vi "Asynchronous - Update Disable Channels.vi"(5 "Channel Data []":T3[](array[typedef])=[{"Labels Settings"=[{"Name"="", "xmlName"="", "Label"=0, "transferPeriod"=0, "SDI_Enabled"=FALSE, "SDI"=0, "Word"={"Param Setting"={"Start Bit"=[], "Num Bits"=[], "Signed?"=[], "ScaleFac"=[], "ScaleOffset"=[], "Block Data Refs"=[], "Encoding"=[], "Values Array"=[], "Item Refs"=[]}}, "TransferType"=enum."ScheduledLabel", "has timestamp?"=FALSE, "Label Disable/Trigger Channel Reference"=0, "Message Handle"=0, "Initialized?"=FALSE, "Word Initial Raw Value"=0, "Label Timestamp Channel Data Reference"=0}], "channel handle"=0, "channel #"=0}] {"Labels Settings"."Label Timestamp Channel Data Reference" format="%.0x"; "Labels Settings"."Label Disable/Trigger Channel Reference" format="%.0x"; "Labels Settings"."Word"."Param Setting"."Item Refs" format="%.0x"; "Labels Settings"."Word"."Param Setting"."Num Bits" min=1 max=32; "Labels Settings"."Word"."Param Setting"."Start Bit" min=8 max=31; "Labels Settings"."Label" format="%.0o"}, 7 "Map":T1[](array[typedef]) {"Channel Data Reference" format="%.0x"}, 8 "Error (in)":errorcluster, 9 "Updated FIFO Index []":i32[](array[numeric]), 10 "Doubles []":dbl[](array[numeric])) -> (0 "Error (out)":errorcluster)   [LabVIEW 2020, in "Ballard Arinc-429 Engine.lvlib"]
uses:
  Ballard Arinc-429 Engine.lvlib
  Shared/Controls and Global/RT HW Channel.ctl
  Shared/Controls and Global/RT Label Settings.ctl
  Shared/Controls and Global/Label.ctl
  Shared/Controls and Global/transferPeriod.ctl
  Shared/Controls and Global/RT Word Settings.ctl
  Shared/Controls and Global/RT Param Setting.ctl
  Shared/Controls and Global/Start Bit.ctl
  Shared/Controls and Global/Number of Bits.ctl
  <vilib>/NI VeriStand/Custom Device API/Block Data Reference.ctl
  <vilib>/NI VeriStand/Custom Device API/Data Reference.ctl
  <vilib>/NI VeriStand/Custom Device API/Custom Device Item Ref.ctl
  Shared/Controls and Global/TransferType.ctl
  RT Controls/RT Tx Association.ctl
  <instrlib>/BTI429Lib/BTI429LV.lvlib
  <vilib>/NI VeriStand/Custom Device Tools/Custom Device Utility Library/Custom Device Utility Library.lvlib
  Shared/Ballard Arinc-429 Shared.lvlib
  <vilib>/NI VeriStand/Custom Device API/Custom Device API.lvlib
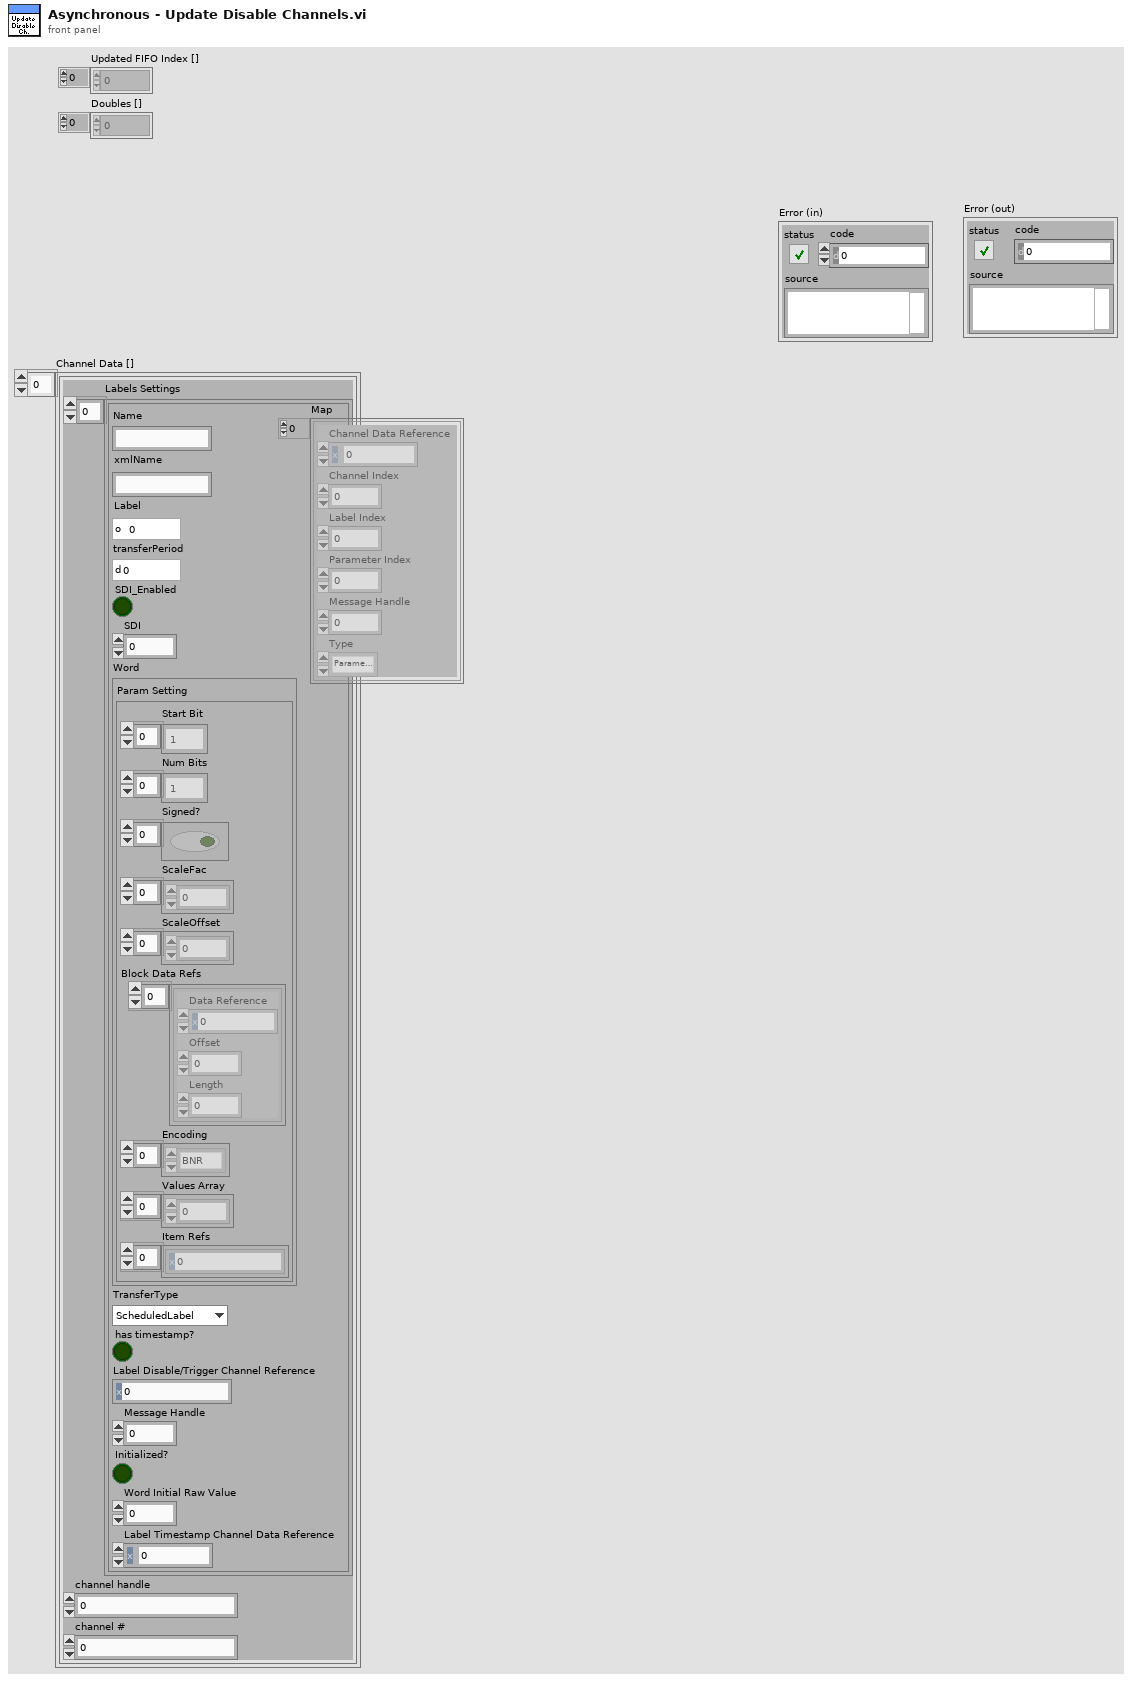
[diagram p1: front panel]
types:
  T1 = typedef "Ballard Arinc-429 Engine.lvlib/RT Tx Association.ctl" = cluster{"Channel Data Reference":T2, "Channel Index":i32, "Label Index":i32, "Parameter Index":i32, "Message Handle":u64, "Type":enum16{"Parameter Channel", "Disable/Trigger Channel"}}
  T2 = typedef "Custom Device API.lvlib/Data Reference.ctl" = i32
  T3 = typedef "Ballard Arinc-429 Shared.lvlib/RT HW Channel.ctl" = cluster{"Labels Settings":T4[], "channel handle":u64, "channel #":u16}
  T4 = typedef "Ballard Arinc-429 Shared.lvlib/RT Label Settings.ctl" = cluster{"Name":string, "xmlName":string, "Label":T5, "transferPeriod":T6, "SDI_Enabled":bool, "SDI":u8, "Word":T7, "TransferType":T13, "has timestamp?":bool, "Label Disable/Trigger Channel Reference":T12, "Message Handle":u64, "Initialized?":bool, "Word Initial Raw Value":u32, "Label Timestamp Channel Data Reference":T2}
  T5 = typedef "Ballard Arinc-429 Shared.lvlib/Label.ctl" = u8
  T6 = typedef "Ballard Arinc-429 Shared.lvlib/transferPeriod.ctl" = u32
  T7 = typedef "Ballard Arinc-429 Shared.lvlib/RT Word Settings.ctl" = cluster{"Param Setting":T8}
  T8 = typedef "Ballard Arinc-429 Shared.lvlib/RT Param Setting.ctl" = cluster{"Start Bit":T9[], "Num Bits":T10[], "Signed?":bool[], "ScaleFac":dbl[], "ScaleOffset":dbl[], "Block Data Refs":T11[], "Encoding":enum16{"BNR", "BCD", "Discrete"}[], "Values Array":dbl[], "Item Refs":T12[]}
  T9 = typedef "Ballard Arinc-429 Shared.lvlib/Start Bit.ctl" = i32
  T10 = typedef "Ballard Arinc-429 Shared.lvlib/Number of Bits.ctl" = i32
  T11 = typedef "Custom Device API.lvlib/Block Data Reference.ctl" = cluster{"Data Reference":T2, "Offset":u64, "Length":u64}
  T12 = typedef "Custom Device API.lvlib/Custom Device Item Ref.ctl" = u64
  T13 = typedef "Ballard Arinc-429 Shared.lvlib/TransferType.ctl" = enum16{"ScheduledLabel", "Acyclic", "Block", "Strobe"}
  T14 = enum16{"Parameter Channel", "Disable/Trigger Channel"}
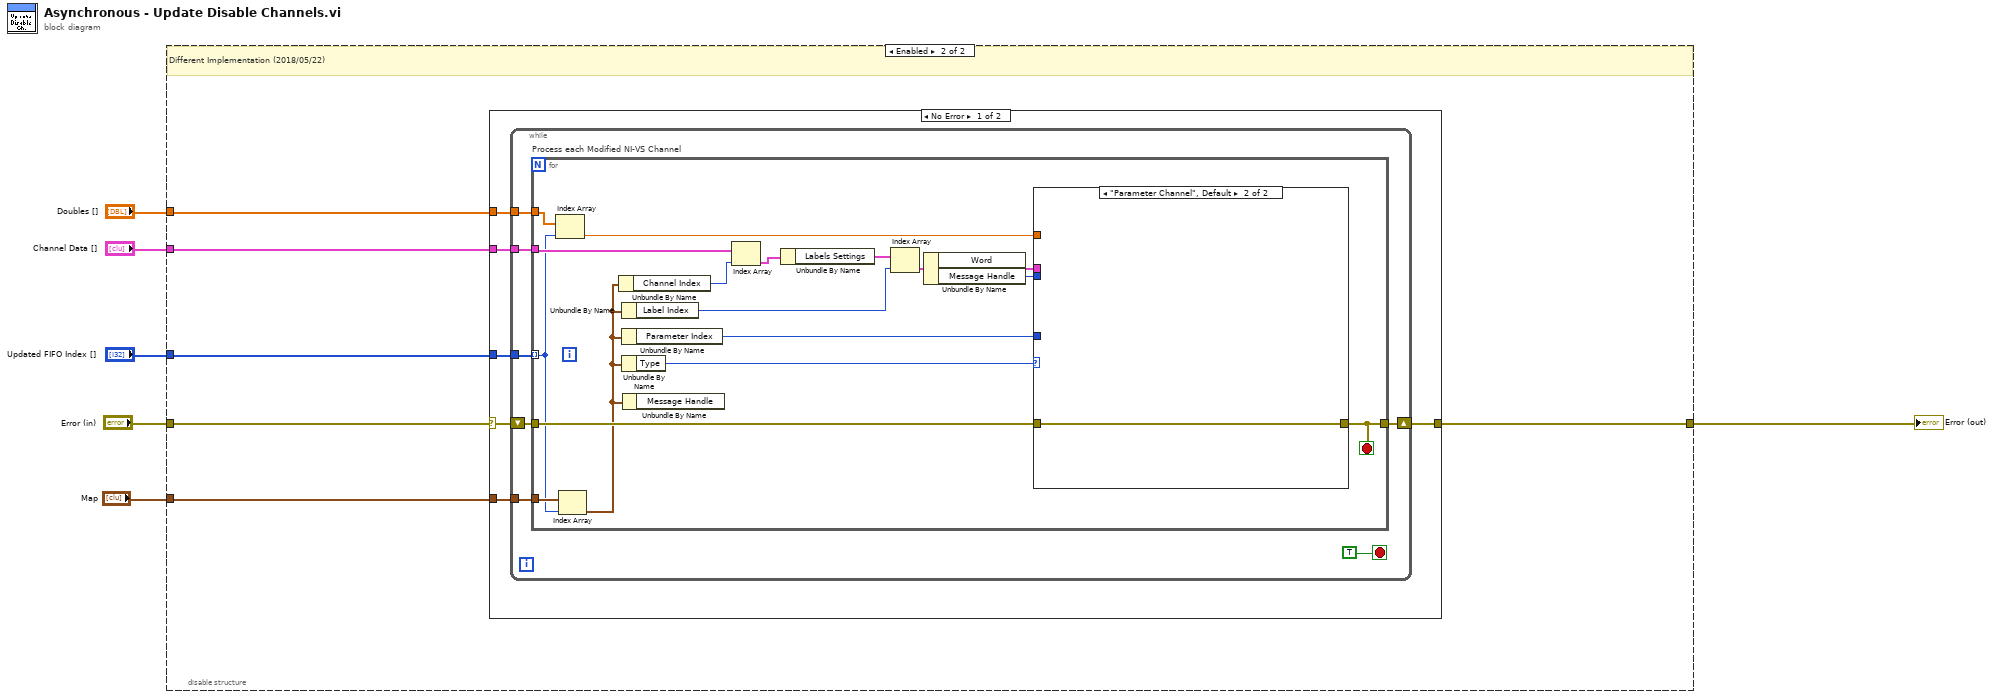
[diagram p0: block diagram]
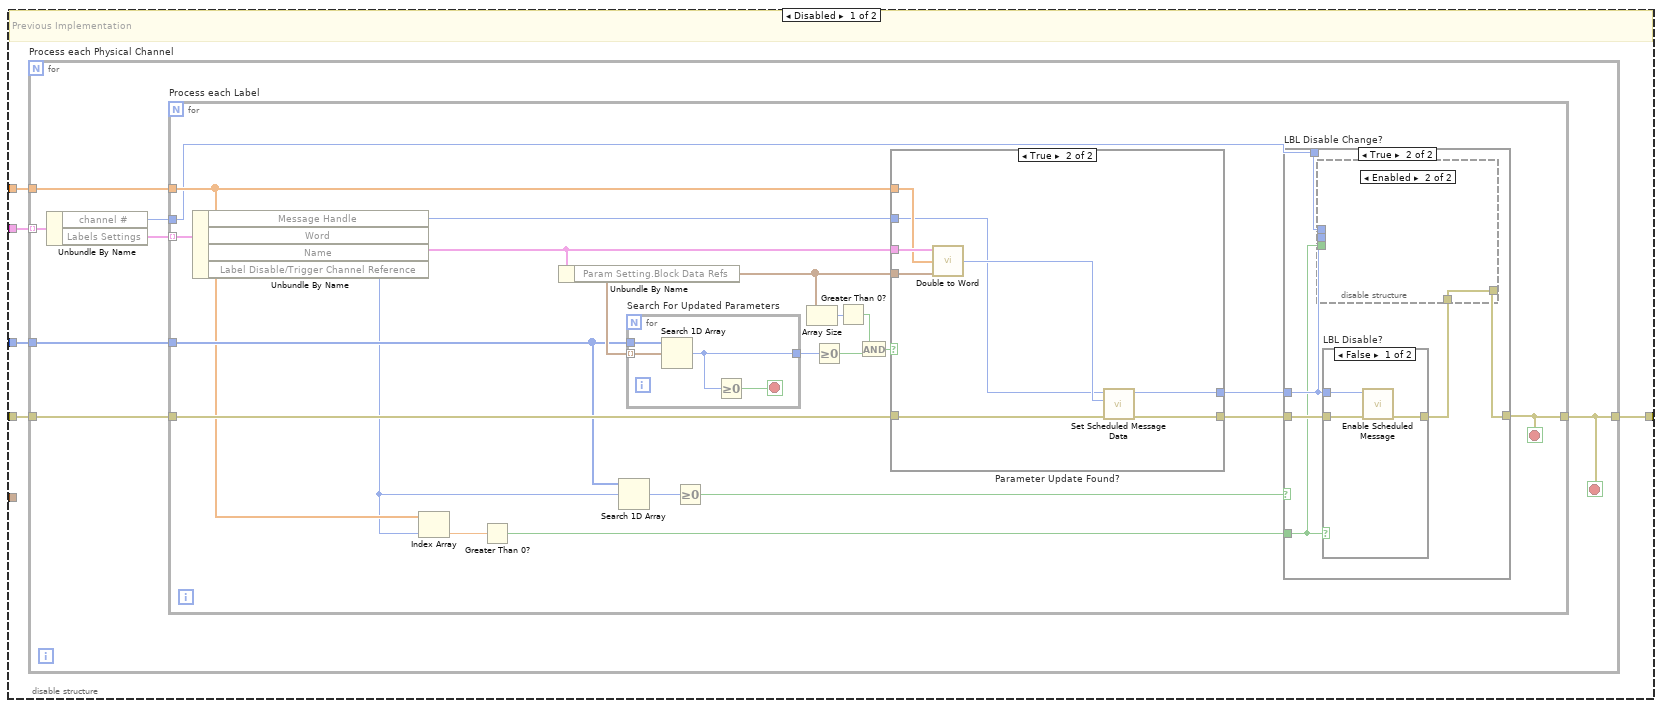
[diagram p2: hidden frame]
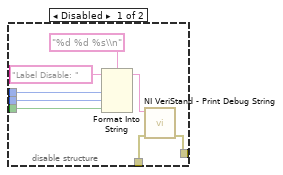
[diagram p4: hidden frame]
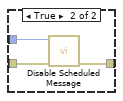
[diagram p5: hidden frame]
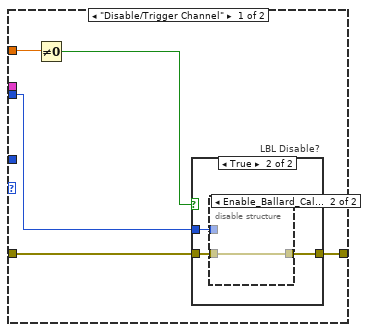
[diagram p7: hidden frame]
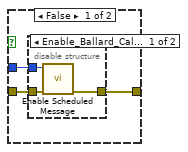
[diagram p8: hidden frame]
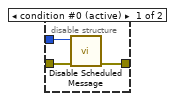
[diagram p10: hidden frame]
diagram:
  n1 = disable-structure shown="Enabled" {
    disable-tunnel: "Channel Data []" -> [w11 w81]
    disable-tunnel: "Updated FIFO Index []" -> [w10 w80]
    disable-tunnel: "Error (in)" -> [w9 w76]
    disable-tunnel: [w8 w79] -> w3
    disable-tunnel: "Doubles []" -> [w7 w78]
    disable-tunnel: "Map" -> [_ w77]
    frame Disabled {
      # "Previous Implementation"
      n2 = for "Process each Physical Channel" {
        tunnel: w11 -> [w18] mode=indexing
        tunnel: w10 -> [w16]
        tunnel: w7 -> [w15]
        tunnel: w9 -> [w14]
        tunnel: [w13] -> w8
        stop <- w13 stop-if-true
        n3 = Unbundle By Name(w18) -> ("channel #"=w12:u16, "Labels Settings"=w17:T4[])
        n4 = for "Process each Label" {
          tunnel: w17 -> [w39] mode=indexing
          tunnel: w16 -> [w31]
          tunnel: w15 -> [w26]
          tunnel: [w28] -> w13
          tunnel: w14 -> [w37]
          tunnel: w12 -> [w20]
          stop <- w28 stop-if-true
          n5 = Unbundle By Name(w39) -> ("Message Handle"=w21:u64, "Word"=w19:T7, "Label Disable/Trigger Channel Reference"=w25:T12)  [unwired: 1 out]
          n6 = Index Array(array=w26, index=w25) -> (element=w24:dbl)
          n7 = Greater Than 0?(x=w24) -> (x > 0?=w23:bool)
          n8 = Unbundle By Name(w19) -> ("Param Setting.Block Data Refs"=w36:T11[])
          n9 = Search 1D Array(1D array=w31, element=w25) -> (index of element=w30:i32)  [unwired: 1 in]
          n10 = for "Search For Updated Parameters" {
            tunnel: w31 -> [w75]
            tunnel: w36 -> [w74] mode=indexing
            tunnel: [w73] -> w38
            stop <- w72 stop-if-true
            n11 = Search 1D Array(1D array=w75, element=w74) -> (index of element=w73:i32)  [unwired: 1 in]
            n12 = Greater Or Equal To 0?(x=w73) -> (x >= 0?=w72:bool)
          }
          n13 = Greater Or Equal To 0?(x=w30) -> (x >= 0?=w29:bool)
          n14 = Array Size(array=w36) -> (size(s)=w35:i32)
          n15 = Greater Or Equal To 0?(x=w38) -> (x >= 0?=w33:bool)
          n16 = Greater Than 0?(x=w35) -> (x > 0?=w34:bool)
          n17 = And(x=w34, y=w33) -> (x .and. y?=w32:bool)
          n18 = case "Parameter Update Found?" shown="True" w32 {
            tunnel: w26 -> [_ w67]
            tunnel: w19 -> [_ w71]
            tunnel: w37 -> [w63 w66]
            tunnel: [w63 w70] -> w27
            tunnel: w36 -> [_ w68]
            tunnel: w21 -> [w62 w65]
            tunnel: [w62 w64] -> w22
            frame False {
            }
            frame True {
              n19 = call "Double to Word.vi"("Word"=w71, "Doubles In []"=w67, "Channel FIFO Buffer Index"=w68) -> ("Word"=w69:u32)  [unwired: 12 in]
              n20 = call <instrlib>:"Set Scheduled Message Data.vi"("error in (no error)"=w66, "value"=w69, "message handle in"=w65) -> ("error out"=w70:errorcluster, "message handle out"=w64:u64)  [unwired: 7 in]
            }
          }
          n21 = case "LBL Disable Change?" shown="True" w29 {
            tunnel: [w40 w45] -> w28
            tunnel: w27 -> [w40 w46]
            tunnel: w23 -> [_ w41]
            tunnel: w22 -> [_ w42]
            tunnel: w20 -> [_ w43]
            frame False {
            }
            frame True {
              n22 = case "LBL Disable?" shown="False" w41 {
                tunnel: [w58 w61] -> w44
                tunnel: w46 -> [w57 w60]
                tunnel: w42 -> [w56 w59]
                frame False {
                  n23 = call <instrlib>:"Enable Scheduled Message.vi"("error in (no error)"=w57, "message handle in"=w56) -> ("error out"=w58:errorcluster)  [unwired: 8 in, 1 out]
                }
                frame True {
                  n24 = call <instrlib>:"Disable Scheduled Message.vi"("error in (no error)"=w60, "message handle in"=w59) -> ("error out"=w61:errorcluster)  [unwired: 8 in, 1 out]
                }
              }
              n25 = disable-structure shown="Enabled" {
                disable-tunnel: [w54 w55] -> w45
                disable-tunnel: w44 -> [w53 w55]
                disable-tunnel: w43 -> [w50 _]
                disable-tunnel: w42 -> [w49 _]
                disable-tunnel: w41 -> [w48 _]
                frame Disabled {
                  n26 = Format Into String(format string="%d %d %s\\n", initial string="Label Disable: ", w50, w49, w48) -> (resulting string=w51:string)  [unwired: 1 in, 1 out]
                  n27 = call <vilib>:"NI VeriStand - Print Debug String.vi"("error in (no error)"=w53, "Message"=w51) -> ("error out"=w54:errorcluster)  [unwired: 9 in]
                }
                frame Enabled {
                }
              }
            }
          }
        }
      }
    }
    frame Enabled {
      # "Different Implementation (2018/05/22)"
      n28 = case shown="No Error" w76 {
        selector: w76 -> [w82 w132]
        tunnel: w81 -> [w87 _]
        tunnel: w80 -> [w86 _]
        tunnel: [w85 w132] -> w79
        tunnel: w78 -> [w84 _]
        tunnel: w77 -> [w83 _]
        frame No Error {
          n29 = while {
            tunnel: w87 -> [w94]
            tunnel: w86 -> [w93]
            tunnel: w84 -> [w90]
            tunnel: w83 -> [w89]
            shift-right: [w91] -> w85
            shift-left: w82 -> [w92]
            stop <- TRUE stop-if-true
            n30 = for "Process each Modified NI-VS Channel" {
              tunnel: w94 -> [w110]
              tunnel: w93 -> [w96] mode=indexing
              tunnel: w90 -> [w98]
              tunnel: w92 -> [w111]
              tunnel: [w99] -> w91
              tunnel: w89 -> [w103]
              stop <- w99 stop-if-true
              n31 = Index Array(array=w98, index=w96) -> (element=w97:dbl)
              n32 = Index Array(array=w103, index=w96) -> (element=w101:T1)
              n33 = Unbundle By Name(w101) -> ("Channel Index"=w109:i32)
              n34 = Unbundle By Name(w101) -> ("Label Index"=w106:i32)
              n35 = Unbundle By Name(w101) -> ("Parameter Index"=w104:i32)
              n36 = Unbundle By Name(w101) -> ("Type"=w100:T14)
              n37 = Unbundle By Name(w101) -> ()  [unwired: 1 out]
              n38 = Index Array(array=w110, index=w109) -> (element=w108:T3)
              n39 = Unbundle By Name(w108) -> ("Labels Settings"=w107:T4[])
              n40 = Index Array(array=w107, index=w106) -> (element=w105:T4)
              n41 = Unbundle By Name(w105) -> ("Word"=w102:T7, "Message Handle"=w95:u64)
              n42 = case shown="\"Parameter Channel\", Default" w100 {
                tunnel: w111 -> [w116 w131]
                tunnel: [w115 w131] -> w99
                tunnel: w104 -> [_ _]
                tunnel: w102 -> [_ _]
                tunnel: w97 -> [w114 _]
                tunnel: w95 -> [w112 _]
                frame "Disable/Trigger Channel" {
                  n43 = Not Equal To 0?(x=w114) -> (x != 0?=w113:bool)
                  n44 = case "LBL Disable?" shown="True" w113 {
                    tunnel: [w119 w126] -> w115
                    tunnel: w116 -> [w118 w125]
                    tunnel: w112 -> [w117 w124]
                    frame False {
                      n45 = disable-structure shown="Enable_Ballard_Calls==True, Default" {
                        disable-tunnel: [w122 w123] -> w119
                        disable-tunnel: w118 -> [w121 w123]
                        disable-tunnel: w117 -> [w120 _]
                        frame condition #0 (active) {
                          n46 = call <instrlib>:"Enable Scheduled Message.vi"("error in (no error)"=w121, "message handle in"=w120) -> ("error out"=w122:errorcluster)  [unwired: 8 in, 1 out]
                        }
                        frame condition #1 {
                        }
                      }
                    }
                    frame True {
                      n47 = disable-structure shown="Enable_Ballard_Calls==False" {
                        disable-tunnel: [w129 w130] -> w126
                        disable-tunnel: w125 -> [w128 w130]
                        disable-tunnel: w124 -> [w127 _]
                        frame condition #0 (active) {
                          n48 = call <instrlib>:"Disable Scheduled Message.vi"("error in (no error)"=w128, "message handle in"=w127) -> ("error out"=w129:errorcluster)  [unwired: 8 in, 1 out]
                        }
                        frame condition #1 {
                        }
                      }
                    }
                  }
                }
                frame "Parameter Channel", Default {
                }
              }
            }
          }
        }
        frame Error {
        }
      }
    }
  }
  "Error (out)" <- w3
